vi "Lin_Rohner_force_sensor.vi"() -> ()   [LabVIEW 2019]
uses:
  <vilib>/Platform/TimedLoop/XDataNode/timing_clust.ctl
  <vilib>/Platform/TimedLoop/XDataNode/nitl_modes.ctl
  <vilib>/Platform/TimedLoop/XDataNode/wakeup.ctl
  <vilib>/Analysis/3filter.llb/Filter Passband Type.ctl
  <vilib>/DAQmx/read.llb/DAQmx Read (Analog 1D DBL NChan 1Samp).vi
  <vilib>/DAQmx/create/channels.llb/DAQmx Create Channel (AI-Voltage-Basic).vi
  <vilib>/DAQmx/miscellaneous.llb/DAQmx Fill In Error Info.vi
  <vilib>/platform/TimedLoop/XDataNode/XDataNode.xnode
  <vilib>/Platform/TimedLoop/XDataNode/XDNodeRunTimeDep.lvlib
  <vilib>/ptbypt/NI_PtbyPt.lvlib
  <vilib>/Analysis/NI_AALBase.lvlib
panel:
  out "Filtered Force sensor [V]":dbl
  out "Filtered Force sensor [V]":dbl(graph)
  in  "filter force sensor":dbl=0.125 format="%0.3f"
  out "Raw Force sensor [V] 2":dbl
  out "Raw Force sensor [V] 2":dbl(graph)
  out "Position":dbl(knob) scale=-32.5..32.5
  out "Filtered Position":dbl
  out "Filtered Postion Graph":dbl(graph)
  in  "stop":bool
  out "Filtered Signal [V]":dbl
  out "Filtered Signal [V]":dbl(graph)
  in  "low cutoff freq: fl 2":dbl=0.125 format="%0.3f"
  out "Raw Hall sensor [V]":dbl(graph)
  out "Raw Hall sensor [V]":dbl
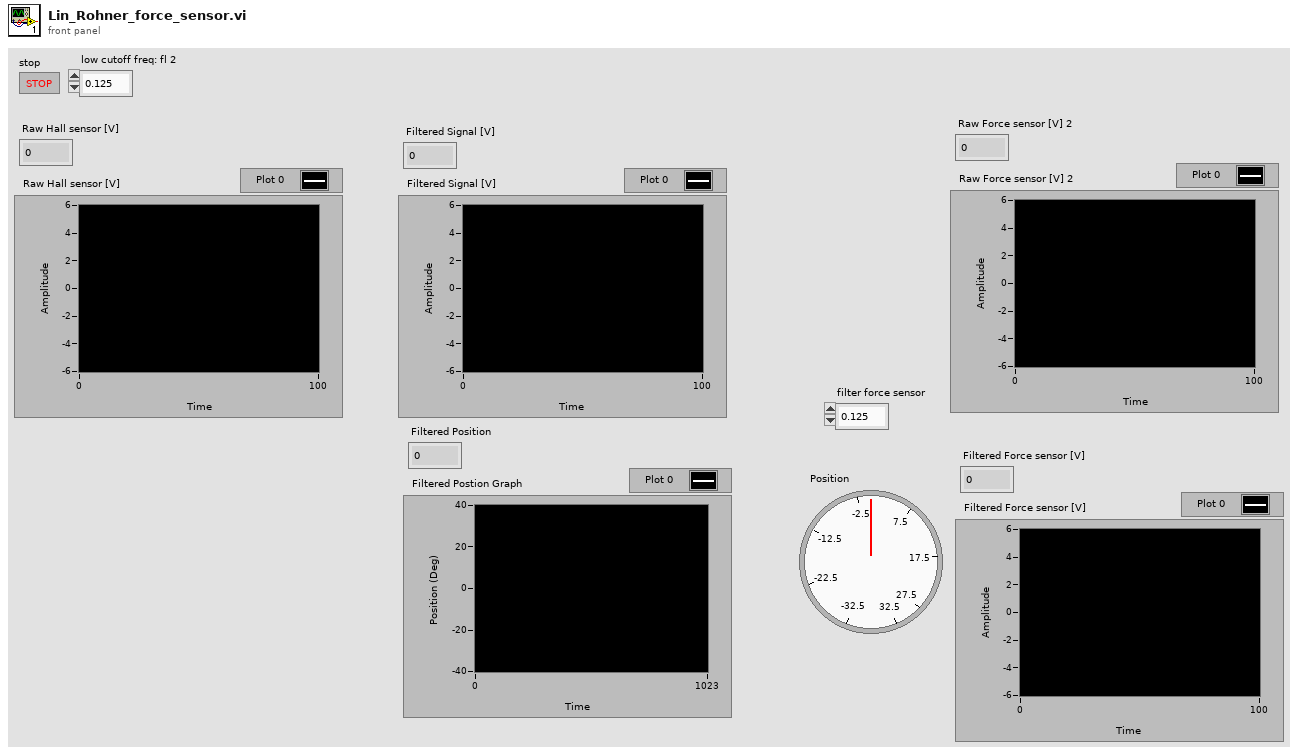
[diagram p1: front panel]
types:
  T1 = typedef "NI_AALBase.lvlib/Filter Passband Type.ctl" = enum32{"Lowpass", "Highpass", "Bandpass", "Bandstop"}
  T2 = typedef "XDNodeRunTimeDep.lvlib/timing_clust.ctl" = cluster{"Expected End [f-1]":u64, "Actual End [f-1]":u64, "Finished Late? [f-1]":bool, "Expected End [i-1]":u64, "Actual End [i-1]":u64, "Finished Late? [i-1]":bool, "Expected Start [i]":u64, "Actual Start [i]":u64, "Expected Start [f]":u64, "Actual Start [f]":u64, "Source Name":string, "Structure Name":string, "Period":i64, "Deadline":i64, "Offset":i64, "Start":i64, "Priority":i32, "Timeout":i32, "Mode":T3, "Wakeup Reason":T4, "Error":errorcluster, "Source Type":string, "Secondary Source Type":string, "Global End Time":u64, "Global Start Time":u64, "Frame Duration":u64, "Iteration Duration":u64, "Assigned CPU":i32, "I/O Scan Engine Mode":u32}
  T3 = typedef "XDNodeRunTimeDep.lvlib/nitl_modes.ctl" = enum32{"No Change", "Process missed periods, maintain original phase", "Discard missed periods, maintain original phase", "Process missed periods, ignore original phase", "Discard missed periods, ignore original phase"}
  T4 = typedef "XDNodeRunTimeDep.lvlib/wakeup.ctl" = enum32{"Normal", "Aborted", "Asynchronous wakeup", "Timing source error", "Timed loop error", "Timeout"}
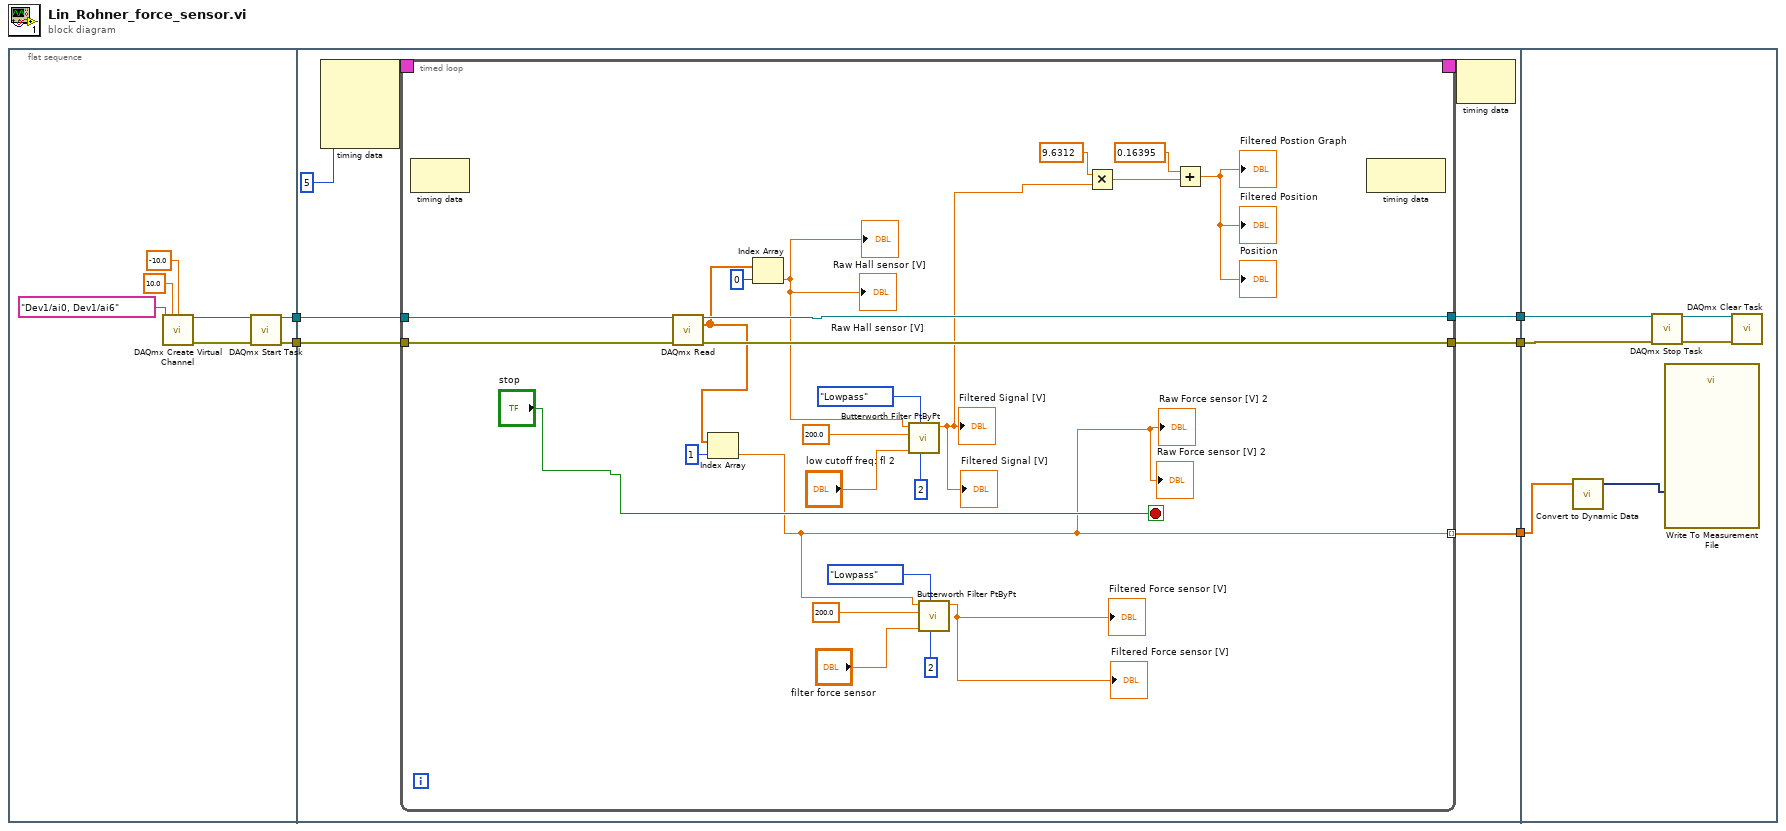
[diagram p0: block diagram]
diagram:
  n1 = flat-sequence {
    tunnel: [w9] -> w5
    tunnel: [w7] -> w3
    tunnel: w5 -> [w18]
    tunnel: [w17] -> w4
    tunnel: w3 -> [w16]
    tunnel: [w15] -> w2
    tunnel: [w13] -> w1
    tunnel: w4 -> [w56]
    tunnel: w2 -> [w54]
    tunnel: w1 -> [w52]
    frame #0 {
      n2 = call-poly <vilib>:"DAQmx Create Virtual Channel.vi"("maximum value"=10.0, "minimum value"=-10.0, "physical channels"=tag "Dev1/ai0, Dev1/ai6") -> ("task out"=w8:refnum<k21>, "error out"=w10:errorcluster)  [unwired: 11 in]
      n3 = call <vilib>:"DAQmx Start Task.vi"("task/channels in"=w8, "error in"=w10) -> ("task out"=w7:refnum<k21>, "error out"=w9:errorcluster)  [unwired: 12 in]
    }
    frame #1 {
      n4 = node-c288(i64 5 ("Period")) -> (w20:T2)  [unwired: 3 in]
      n5 = timed-loop {
        timing: w20 -> [_]
        timing-out: [_] -> w19
        tunnel: w18 -> [w44]
        tunnel: [w43] -> w17
        tunnel: w16 -> [w39]
        tunnel: [w38] -> w15
        tunnel: [w21] -> w13 mode=indexing
        stop <- "stop" stop-if-true
        n6 = node-c288() -> ()  [unwired: 1 in, 1 out]
        n7 = call-poly <vilib>:"DAQmx Read.vi"("task/channels in"=w39, "error in"=w44) -> ("task out"=w38:refnum<k21>, "data"=w27:dbl[], "error out"=w43:errorcluster)  [unwired: 11 in]
        n8 = Index Array(array=w27, index=1) -> (element=w21:dbl)
        "Raw Force sensor [V] 2" <- w21
        "Raw Force sensor [V] 2" <- w21
        n9 = Index Array(array=w27, index=0) -> (element=w29:dbl)
        "Raw Hall sensor [V]" <- w29
        "Raw Hall sensor [V]" <- w29
        n10 = call <vilib>:"Butterworth Filter PtByPt.vi"("order"=2, "filter type"=Filter_Passband_Type."Lowpass", "low cutoff freq: fl"="low cutoff freq: fl 2", "sampling freq: fs"=200.0, "x"=w29) -> ("Filtered x"=w31:dbl)  [unwired: 4 in, 1 out]
        "Filtered Signal [V]" <- w31
        "Filtered Signal [V]" <- w31
        n11 = call <vilib>:"Butterworth Filter PtByPt.vi"("order"=2, "filter type"=Filter_Passband_Type."Lowpass", "low cutoff freq: fl"="filter force sensor", "sampling freq: fs"=200.0, "x"=w21) -> ("Filtered x"=→"Filtered Force sensor [V]" →"Filtered Force sensor [V]":dbl)  [unwired: 4 in, 1 out]
        n12 = Multiply(x=9.6312, y=w31) -> (x*y=w34:dbl)
        n13 = Add(x=0.16395, y=w34) -> (x+y=→"Filtered Postion Graph" →"Filtered Position" →"Position":dbl)
        n14 = node-c288() -> ()  [unwired: 1 in, 1 out]
      }
      n15 = node-c288(w19) -> ()  [unwired: 1 out]
    }
    frame #2 {
      n16 = call "Convert to Dynamic Data"("Array"=w52) -> ("Dynamic Data Type"=w51:dynamicdata)  [unwired: 3 in]
      n17 = call <vilib>:"DAQmx Stop Task.vi"("task/channels in"=w54, "error in"=w56) -> ("task out"=w53:refnum<k21>, "error out"=w55:errorcluster)  [unwired: 12 in]
      n18 = call "Write To Measurement File"("Signals"=w51) -> ()  [unwired: 16 in, 3 out]
      n19 = call <vilib>:"DAQmx Clear Task.vi"("task in"=w53, "error in"=w55) -> ()  [unwired: 13 in, 1 out]
    }
  }
